vi "Read Imagesdata from single TDMS.vi"(8 "Experiment Parameters":T1, 9 "Current Plane":i32, 10 "Channel":i32=1, 11 "Current Trial TDMS Ref":refnum<k34>) -> (1 "Ref Image Array":dbl[][](array[numeric]), 3 "Image Array":i16[][][](array[numeric]))   [LabVIEW 2017]
uses:
  Typedefs/Experiment Parameters.ctl
panel:
  out "Array 2":i32[](array[numeric])
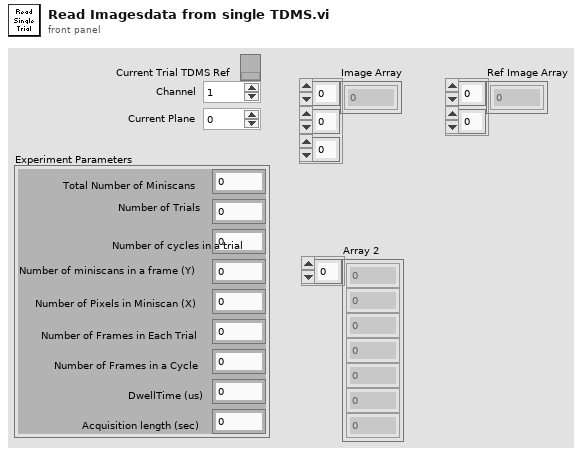
[diagram p1: front panel]
types:
  T1 = typedef "Experiment Parameters.ctl" = cluster{"Total Number of Miniscans":i32, "Number of Trials":i32, "Number of cycles in a trial":i32, "Number of miniscans in a frame (Y)":i32, "Number of Pixels in Miniscan (X)":i32, "Number of Frames in Each Trial":i32, "Number of Frames in a Cycle":i32, "DwellTime (us)":dbl, "Acquisition length (sec)":dbl}
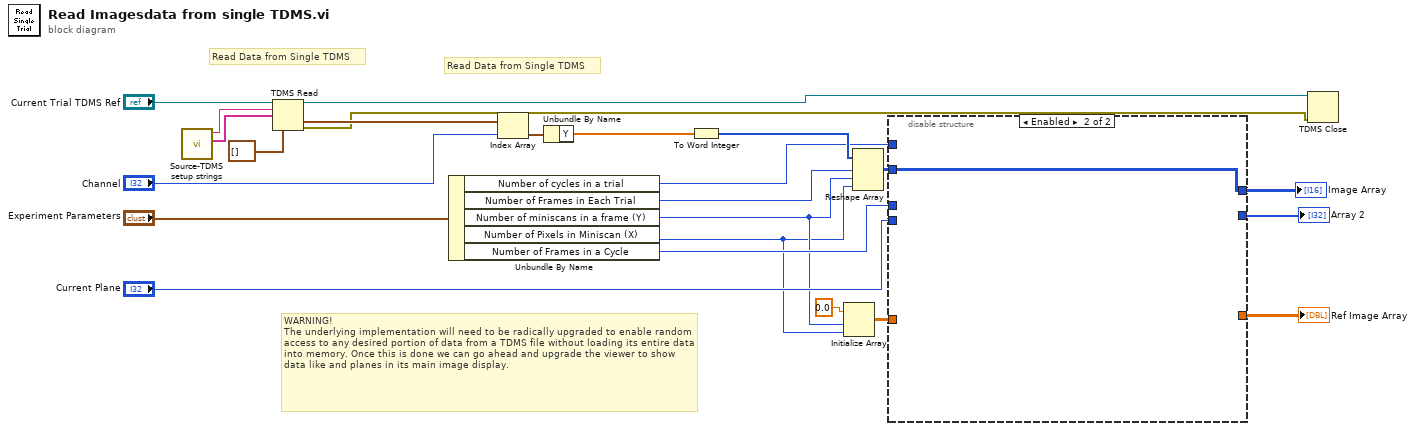
[diagram p0: block diagram]
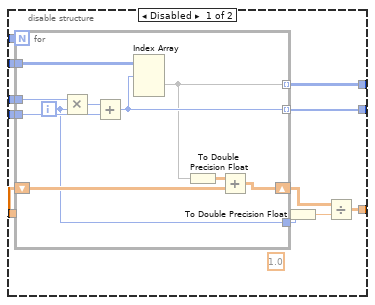
[diagram p2: hidden frame]
diagram:
  # "WARNING!\nThe underlying implementation will need to be radically upgraded to enable random access to any desired portion of data from a TDMS file without loading its entire data into memory. Once this is done we can go ahead and upgrade the viewer to show data like and planes in its main image display."
  # "Read Data from Single TDMS"
  # "Read Data from Single TDMS"
  n1 = call "Source-TDMS setup strings.vi"() -> ("Functional imaging TDMS channel names array"=w20:string[], "TDMS group name"=w21:string)  [unwired: 10 in]
  n2 = TDMS Read(0:"Current Trial TDMS Ref", 5:w21, 7:w20, 12:waveform(dbl)[] [] ("data type")) -> (4:w2:refnum<k34>, 10:w22:waveform(dbl)[], 15:w1:errorcluster)  [unwired: 4 in, 3 out]
  n3 = Unbundle By Name("Experiment Parameters") -> ("Number of cycles in a trial"=w13:i32, "Number of Frames in Each Trial"=w12:i32, "Number of miniscans in a frame (Y)"=w7:i32, "Number of Pixels in Miniscan (X)"=w3:i32, "Number of Frames in a Cycle"=w10:i32)
  n4 = Index Array(array=w22, index="Channel") -> (element=w23:waveform(dbl))
  n5 = Unbundle By Name(w23) -> ("Y"=w24:dbl[])
  n6 = To Word Integer(number=w24) -> (16bit integer=w18:i16[])
  n7 = Initialize Array(0.0, w7, w3) -> (w5:dbl[][])
  n8 = Reshape Array(w18, w12, w7, w3) -> (w17:i16[][][])
  n9 = disable-structure shown="Enabled" {
    disable-tunnel: w17 -> [w35 w46]
    disable-tunnel: [w34 w46] -> w16
    disable-tunnel: [w33 _] -> w14
    disable-tunnel: w13 -> [w32 _]
    disable-tunnel: w10 -> [w31 _]
    disable-tunnel: "Current Plane" -> [w30 _]
    disable-tunnel: w5 -> [w29 _]
    disable-tunnel: [w25 _] -> w4
    frame Disabled {
      (unwired) 1.0 ("double precision float")
      n10 = for {
        N: w32 -> [_]
        tunnel: w35 -> [w41]
        tunnel: [w40] -> w34 mode=indexing
        tunnel: [w45] -> w33 mode=indexing
        tunnel: w31 -> [w43]
        tunnel: w30 -> [w42]
        shift-right: [w38] -> w28
        shift-left: w29 -> [w37]
        tunnel: [w36] -> w27
        i -> [w36]
        n11 = Multiply(x=w43, y=w36) -> (x*y=w44:i32)
        n12 = Add(x=w44, y=w42) -> (x+y=w45:i32)
        n13 = Index Array(array=w41, index (dim 0)=w45) -> (element=w40:i16[][])  [unwired: 2 in]
        n14 = To Double Precision Float(number=w40) -> (double precision float=w39:dbl[][])
        n15 = Add(x=w39, y=w37) -> (x+y=w38:dbl[][])
      }
      n16 = To Double Precision Float(number=w27) -> (double precision float=w26:dbl)
      n17 = Divide(x=w28, y=w26) -> (x/y=w25:dbl[][])
    }
    frame Enabled {
    }
  }
  "Image Array" <- w16
  "Array 2" <- w14
  "Ref Image Array" <- w4
  n18 = TDMS Close(8:w1, 11:w2) -> ()  [unwired: 2 out]
